vi "SetRootPath.vi"(8 "error in (no error)":errorcluster, 9 "Root path":path, 11 "IExporter in":refnum<class "IExporter.lvclass">) -> (0 "error out":errorcluster, 3 "IExporter out":refnum<class "IExporter.lvclass">)   [LabVIEW 2020, in "ExtensionInterfaces.lvlib" / "IExporter.lvclass"]
uses:
  IExporter.lvclass
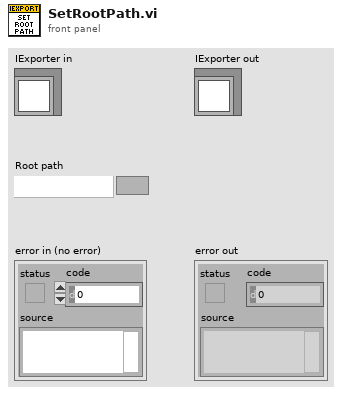
[diagram p1: front panel]
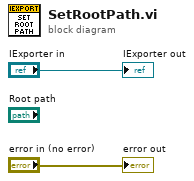
[diagram p0: block diagram]
diagram:
  "error out" <- "error in (no error)"
  "IExporter out" <- "IExporter in"
